vi "Test--temp.vi"() -> ()   [LabVIEW 2024, in "Flexi-Flow Modbus TCP API.lvlib"]
uses:
  Flexi-Flow Modbus TCP API.lvlib
  ca-ec-test-stand/Dependencies/gmodbustcp-main/Sources/Lvlib/ModBusVIEWoTCP.lvlib
panel:
  in  "Type":u16
  out "Words 2":i16[](array[numeric])
  out "Words":i16[](array[numeric])
  out "Bits 2":bool[](array[boolean])
  in  "Quantity of bits (1)":u16=1
  in  "Bit address":u16
  in  "Unit identifier (x1)":u8=1
  out "Bits":bool[](array[boolean])
  out "Information out":T1 {"Unit identifier" max=247; "exceptionCode" max=247}
  in  "Network":T2={"server address"="192.168.100.10", "remote port (502)"=502}
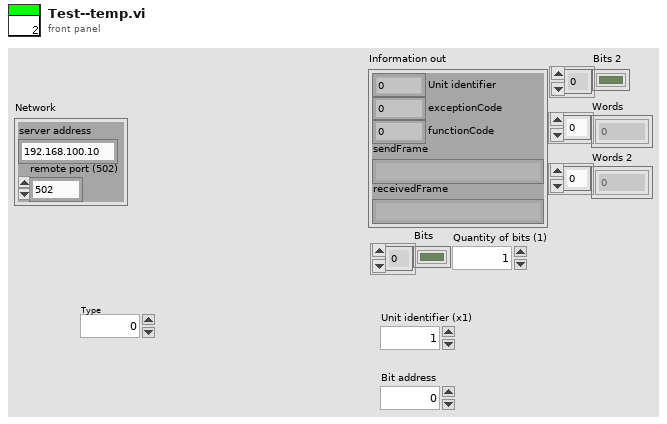
[diagram p1: front panel]
types:
  T1 = cluster{"Unit identifier":u8, "exceptionCode":u8, "functionCode":u8, "sendFrame":string, "receivedFrame":string}
  T2 = cluster{"server address":string, "remote port (502)":u16}
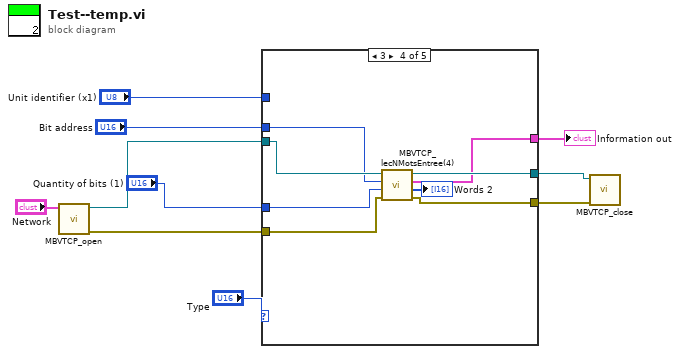
[diagram p0: block diagram]
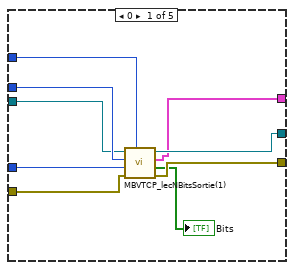
[diagram p2: hidden frame]
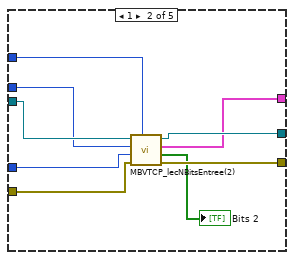
[diagram p3: hidden frame]
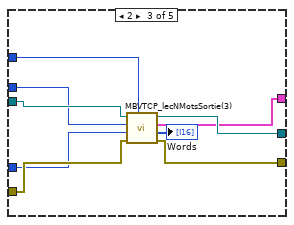
[diagram p4: hidden frame]
diagram:
  n1 = call "MBVTCP_open.vi"("Network"="Network") -> ("error out"=w6:errorcluster, "NetRefTCP out"=w7:refnum<k5>)  [unwired: 2 in, 7 out]
  n2 = case shown="3" "Type" {
    tunnel: "Bit address" -> [w19 w22 w31 w40 _]
    tunnel: w7 -> [w18 w28 w37 w45 w47]
    tunnel: w6 -> [w16 w25 w34 w44 w46]
    tunnel: [w17 w27 w36 w43 w47] -> w5
    tunnel: [w15 w24 w33 w42 w46] -> w4
    tunnel: [w14 w26 w35 w41 _] -> w3
    tunnel: "Unit identifier (x1)" -> [w12 w23 w32 _ _]
    tunnel: "Quantity of bits (1)" -> [w11 w21 w30 w38 _]
    frame 0 {
      n3 = call "MBVTCP_lecNBitsSortie(1).vi"("Unit identifier (x1)"=w12, "error in"=w16, "Quantity of bits (1)"=w11, "Bit address"=w19, "NetRefTCP in"=w18) -> ("error out"=w15:errorcluster, "Bits"=→"Bits":bool[], "Information out"=w14:T1, "NetRefTCP out"=w17:refnum<k5>)  [unwired: 1 in, 2 out]
    }
    frame 1 {
      n4 = call "MBVTCP_lecNBitsEntree(2).vi"("Unit identifier (x1)"=w23, "error in"=w25, "Quantity of bits (1)"=w21, "Bit address"=w22, "NetRefTCP in"=w28) -> ("error out"=w24:errorcluster, "Bits"=→"Bits 2":bool[], "Information out"=w26:T1, "NetRefTCP out"=w27:refnum<k5>)  [unwired: 1 in, 2 out]
    }
    frame 2 {
      n5 = call "MBVTCP_lecNMotsSortie(3).vi"("Unit identifier (x1)"=w32, "error in"=w34, "Quantity of words (1)"=w30, "Word address"=w31, "NetRefTCP in"=w37) -> ("error out"=w33:errorcluster, "Words"=→"Words":i16[], "Information out"=w35:T1, "NetRefTCP out"=w36:refnum<k5>)  [unwired: 1 in, 2 out]
    }
    frame 3 {
      n6 = call "MBVTCP_lecNMotsEntree(4).vi"("error in"=w44, "Quantity of words (1)"=w38, "Word address"=w40, "NetRefTCP in"=w45) -> ("error out"=w42:errorcluster, "Words"=→"Words 2":i16[], "Information out"=w41:T1, "NetRefTCP out"=w43:refnum<k5>)  [unwired: 1 in, 3 out]
    }
    frame Default {
    }
  }
  "Information out" <- w3
  n7 = call "MBVTCP_close.vi"("error in"=w4, "NetRefTCP in"=w5) -> ()  [unwired: 10 out]
